vi "VI Properties Editor.vi"() -> ()   [LabVIEW 2023, in "VI Properties Editor.lvlib"]
doc: "Displays a window to add and edit properties of VIs in a streamlined way."
uses:
  VI Properties Editor.lvlib
  Tree Map/Tree Map/Tree Map.lvclass
  <vilib>/picture/picture.llb/imagedata.ctl
  CTLs/Main State Data.ctl
  CTLs/Control Properties.ctl
  CTLs/VI Properties.ctl
  CTLs/Main Front Panel Controls.ctl
  CTLs/Config.ctl
  <vilib>/Utility/miscctls.llb/LVSelectionTypeDef.ctl
  CTLs/Filter Type.ctl
  CTLs/Column Name.ctl
  CTLs/Filter Info.ctl
  CTLs/Confirmation Type.ctl
  CTLs/Main References.ctl
  CTLs/Sort Info.ctl
  CTLs/VI Data Map.ctl
  <vilib>/Utility/miscctls.llb/LVRowAndColumnTypeDef.ctl
  <vilib>/Utility/miscctls.llb/LVNodeAndColumnTypeDef.ctl
panel:
  in  "VI Tree":string(tree) caption="Select a VI to View/Edit Properties:"
  in  "Same Title as VI?":bool caption="Same as VI name"
  in  "Window Title":string
  in  "Add Copyright":bool
  out "Inline?":bool
  out "Reentrant?":bool
  in  "Set all VIs":bool
  in  "Help Tag":string
  in  "Help Path":string
  out "Path to VI":string
  in  "VI Description":string
  out "VI Connector Pane":picture
  in  "Controls":string[][](table)
  out "Current Filter":string
  out "Current Counts":string
  out "Current Source":string
  # "Controls"
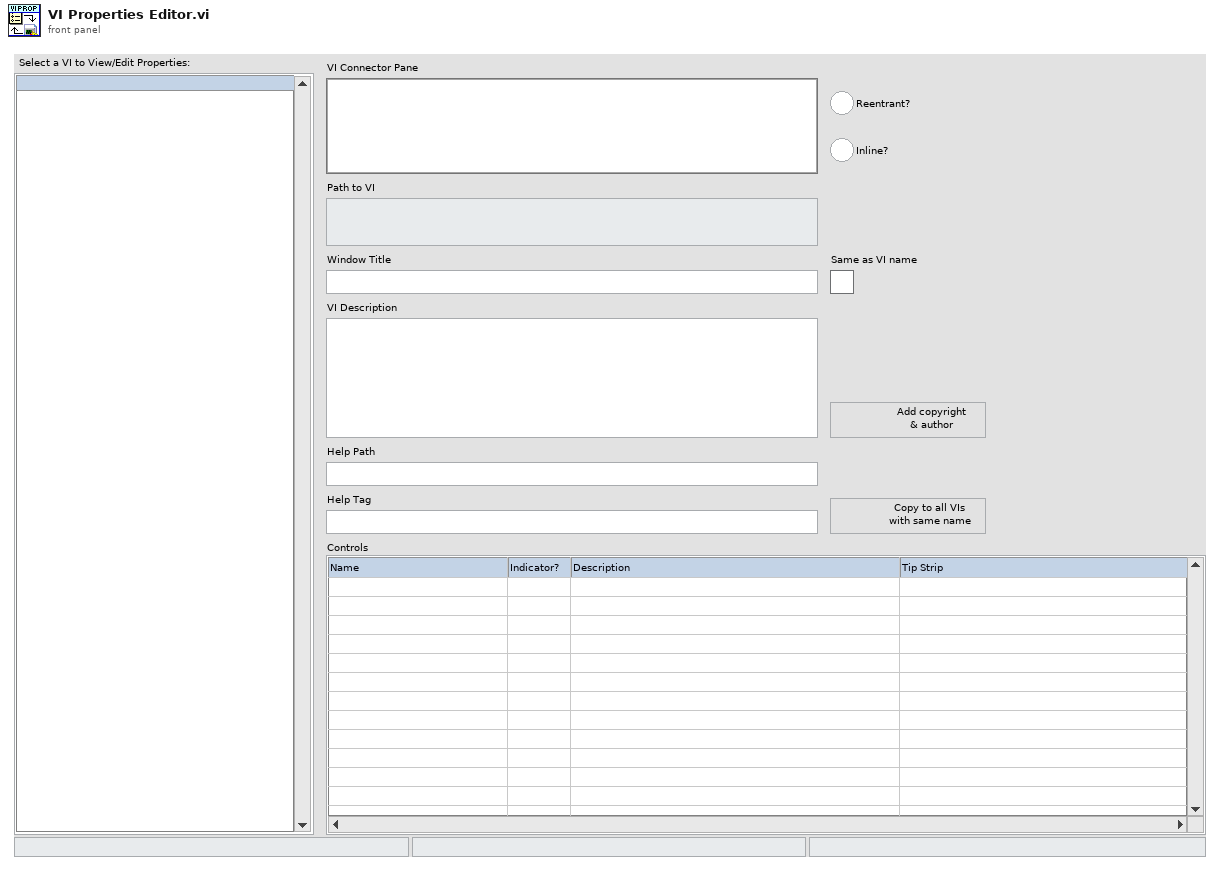
[diagram p1: front panel]
types:
  T1 = typedef "VI Properties Editor.lvlib/Main State Data.ctl" = cluster{"Core":cluster{"Current VI Reference":refnum<vi>, "Close Panel on Exit?":bool}, "FP Refs":T2, "New VI Data":T3, "Saved VI Data":T3, "Current Path":path, "FP":T7, "Config Path":path, "Config":T8, "Desc Selection":T12, "Displayed Hierarchies":string[], "Filter":T9, "Sort":T13, "Tree Map":refnum<class "Tree Map.lvclass">}
  T2 = typedef "VI Properties Editor.lvlib/Main References.ctl" = cluster{"VI Tree":refnum<vi>, "Window Title":refnum<vi>, "Same as VI?":refnum<vi>, "VI Desc":refnum<vi>, "Help Path":refnum<vi>, "Help Tag":refnum<vi>, "Controls":refnum<vi>}
  T3 = typedef "VI Properties Editor.lvlib/VI Data Map.ctl" = map{string, cluster{"VI":T4, "Ctl Properties":T6[]}}
  T4 = typedef "VI Properties Editor.lvlib/VI Properties.ctl" = cluster{"Name":string, "Path":path, "Type":enum32{"invalid VI type", "Standard VI", "Control VI", "Global VI", "Polymorphic VI", "Configuration VI", "SubSystem", "Facade VI", "Method VI", "Statechart Diagram VI"}, "Window Title":string, "Description":string, "Help Path":path, "Help Tag":string, "Custom Title?":bool, "Reentrant?":bool, "Inlined?":bool, "Conpane Img":T5}
  T5 = typedef "imagedata.ctl" = cluster{"image type":i32, "image depth":i32, "image":u8[], "mask":u8[], "colors":u32[], "Rectangle":cluster{"left":i16, "top":i16, "right":i16, "bottom":i16}}
  T6 = typedef "VI Properties Editor.lvlib/Control Properties.ctl" = cluster{"UID":i32, "Name":string, "Description":string, "Tip Strip":string, "Is Indicator?":bool, "Is on ConPane?":bool}
  T7 = typedef "VI Properties Editor.lvlib/Main Front Panel Controls.ctl" = cluster{"VI Selected":string, "Help Path":string, "Help Tag":string, "VI Desc":string, "Controls":string[][], "Window Title":string, "Same Title?":bool}
  T8 = typedef "VI Properties Editor.lvlib/Config.ctl" = cluster{"Copyright Path":path, "Recent Folders":path[], "Recent Files":path[], "Recent Filters":T9[], "Abbreviate Names?":bool, "Format Bold Tags?":bool, "Show ConPane Only?":bool, "Confirm Save?":bool, "Confirm Revert?":bool, "Confirm Save All?":bool, "Confirm Revert All?":bool, "Confirm Exit?":bool}
  T9 = typedef "VI Properties Editor.lvlib/Filter Info.ctl" = cluster{"Filter Column":T10, "Filter Type":T11, "Filter Value":string, "New Data?":bool, "Enabled?":bool}
  T10 = typedef "VI Properties Editor.lvlib/Column Name.ctl" = enum16{"Name", "Path", "Type", "Window Title", "Description", "Help Path", "Help Tag", "Custom Title?", "Reentrant?", "Inlined?"}
  T11 = typedef "VI Properties Editor.lvlib/Filter Type.ctl" = enum16{"Contains", "Equals", "Starts with", "Ends with", "Does not contain", "Does not equal", "Is empty", "Is not empty"}
  T12 = typedef "LVSelectionTypeDef.ctl" = cluster{"Selection Start":u32, "Selection End":u32}
  T13 = typedef "VI Properties Editor.lvlib/Sort Info.ctl" = cluster{"Sort Column":T10, "Ascending?":bool, "Enabled?":bool}
  T14 = enum32{"Invalid", "Standard", "Closed", "Hidden", "Minimized", "Maximized"}
  T15 = enum32{"invalid app kind", "Development System", "Run Time System", "Student Edition", "Embedded LabVIEW", "Evaluation", "Custom"}
  T16 = typedef "LVRowAndColumnTypeDef.ctl" = cluster{"Row":i32, "Column":i32}
  T17 = enum32{"invalid VI type", "Standard VI", "Control VI", "Global VI", "Polymorphic VI", "Configuration VI", "SubSystem", "Facade VI", "Method VI", "Statechart Diagram VI"}
  T18 = typedef "VI Properties Editor.lvlib/Confirmation Type.ctl" = enum16{"Save", "Revert", "Save All", "Revert All"}
  T19 = typedef "LVNodeAndColumnTypeDef.ctl" = cluster{"Node":string, "Column":i32}
  T20 = map{string, cluster{"VI":T4, "Ctl Properties":T6[]}}
  T21 = enum8{"Enabled", "Disabled", "Disabled and Grayed Out"}
  T22 = enum16{"Left Button", "Center Button", "Right Button", "Window Close"}
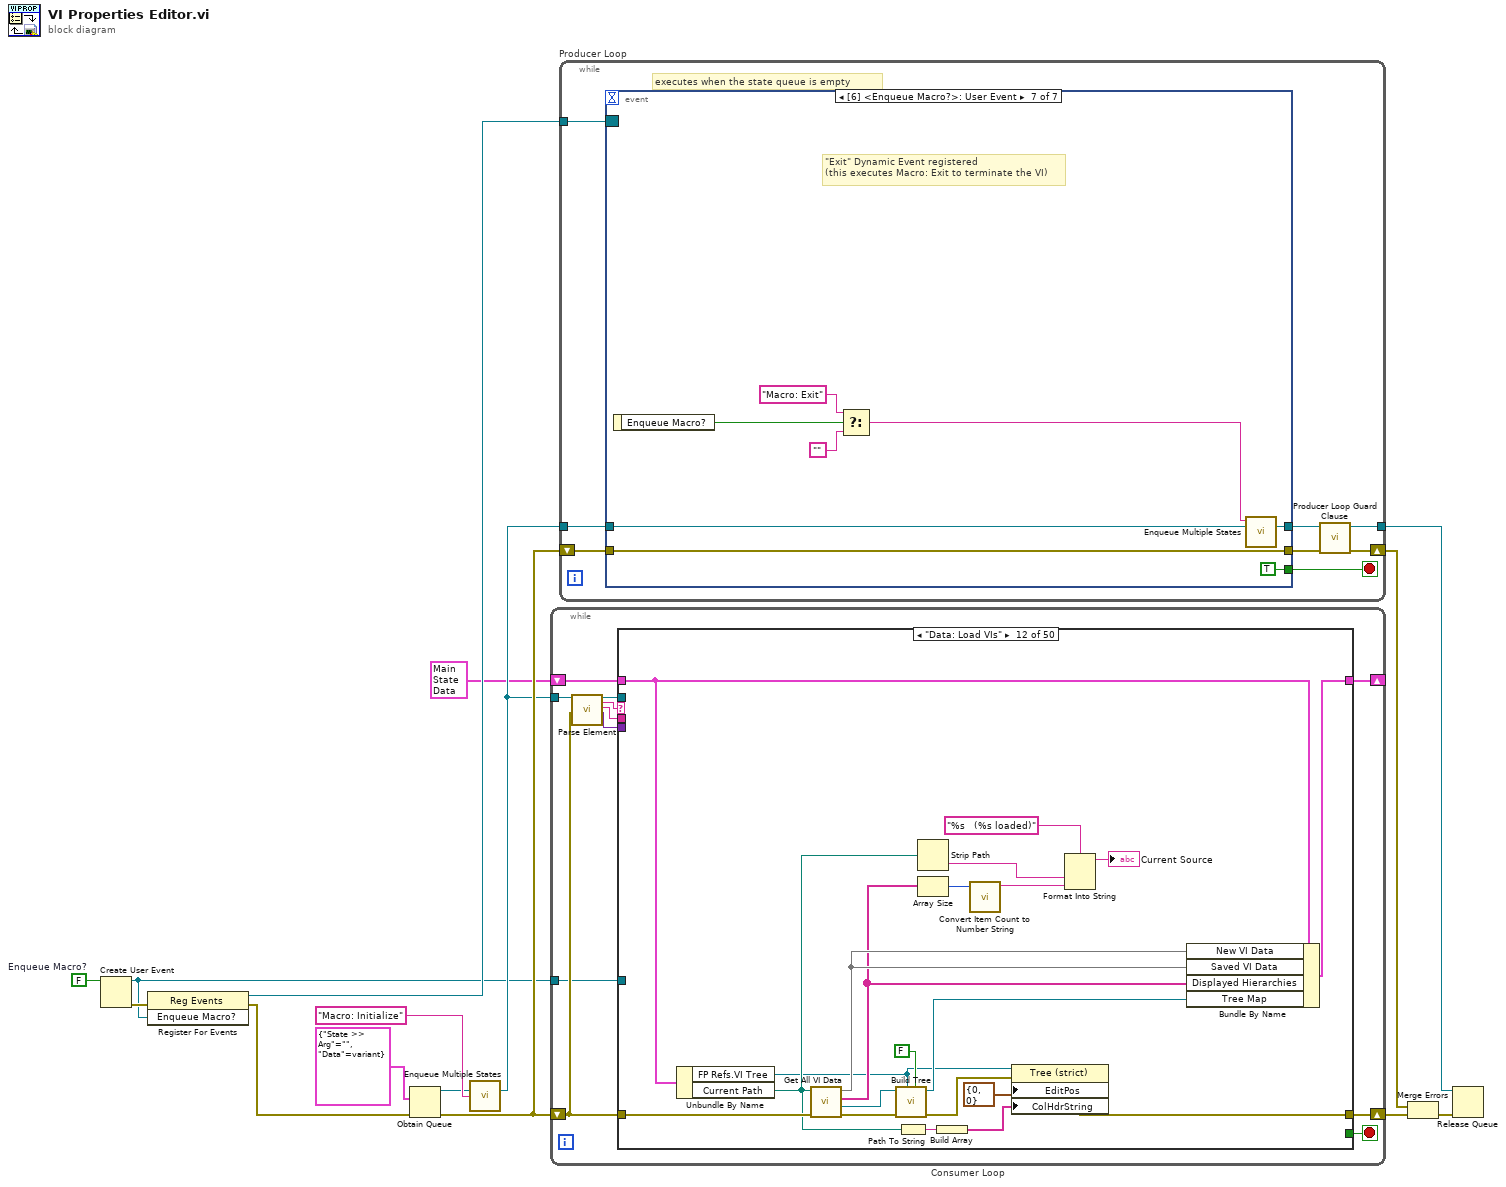
[diagram p0: block diagram]
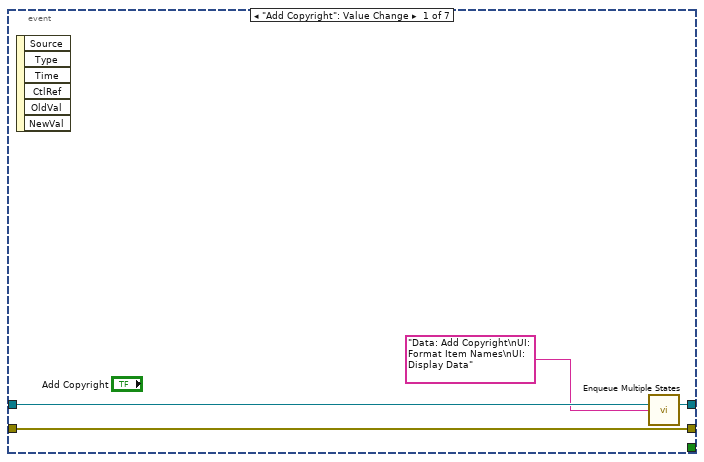
[diagram p2: hidden frame]
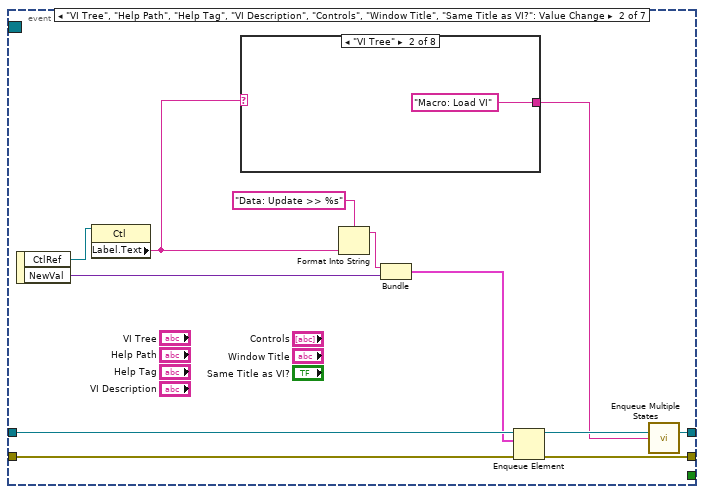
[diagram p3: hidden frame]
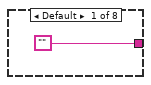
[diagram p4: hidden frame]
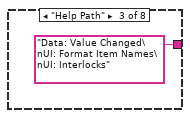
[diagram p5: hidden frame]
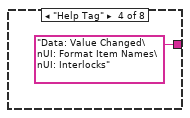
[diagram p6: hidden frame]
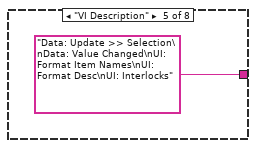
[diagram p7: hidden frame]
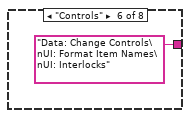
[diagram p8: hidden frame]
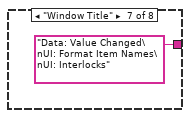
[diagram p9: hidden frame]
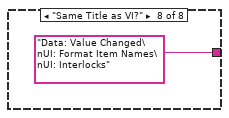
[diagram p10: hidden frame]
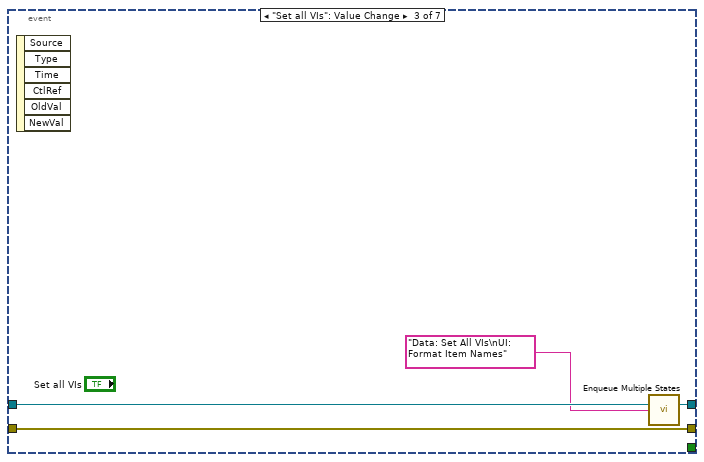
[diagram p11: hidden frame]
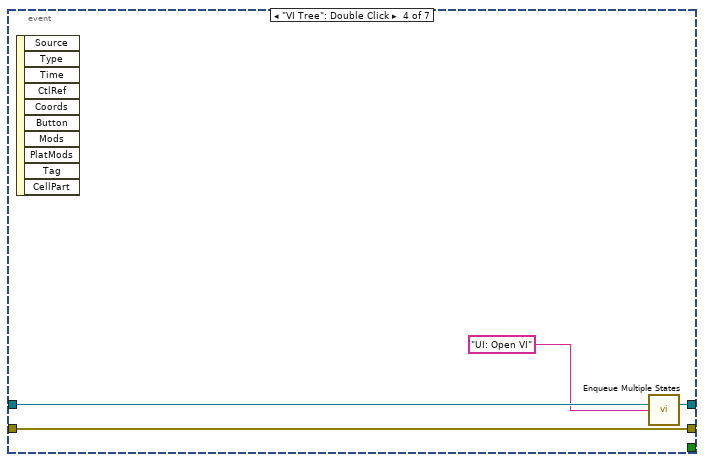
[diagram p12: hidden frame]
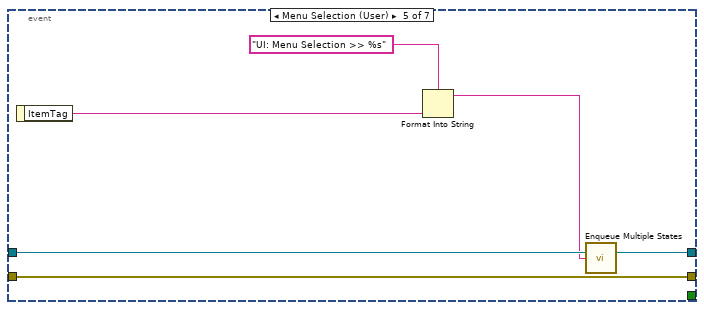
[diagram p13: hidden frame]
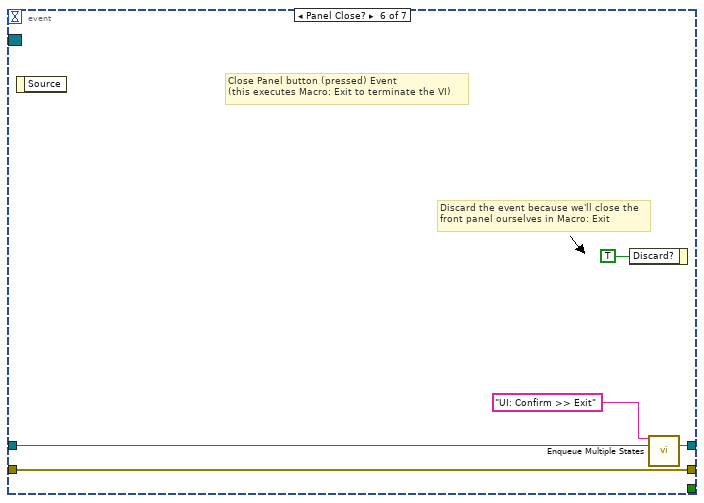
[diagram p14: hidden frame]
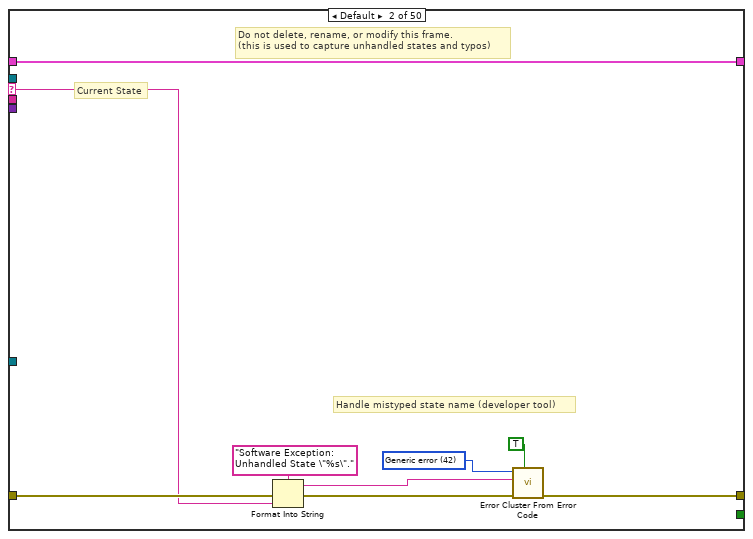
[diagram p16: hidden frame]
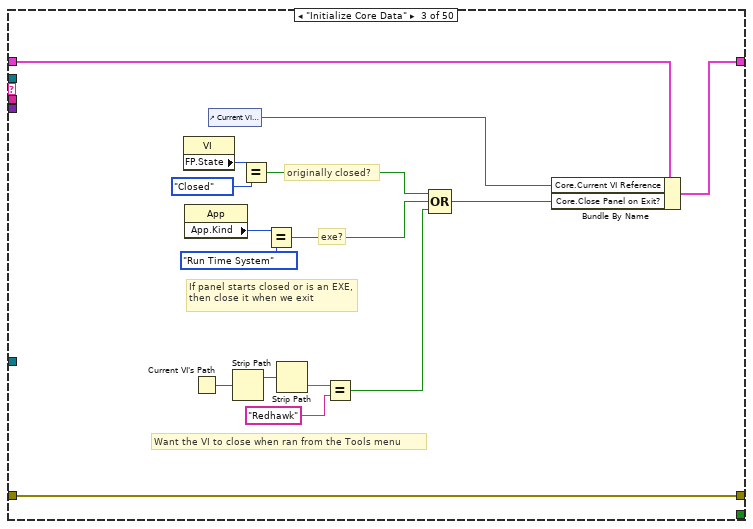
[diagram p17: hidden frame]
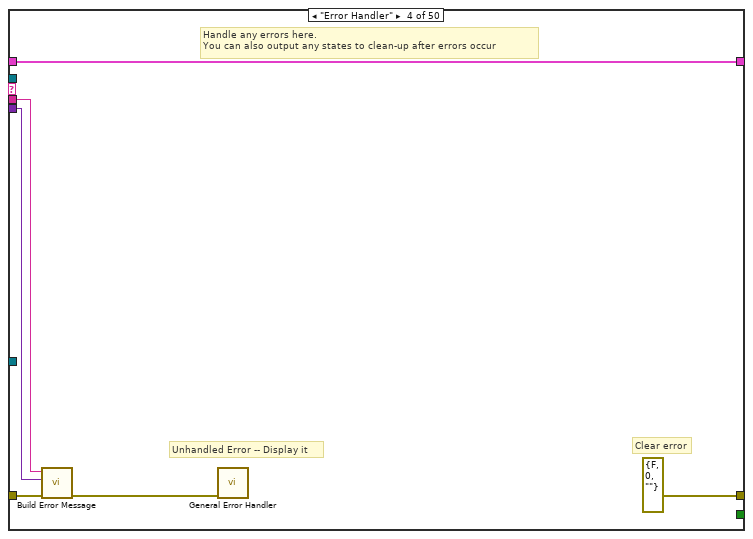
[diagram p18: hidden frame]
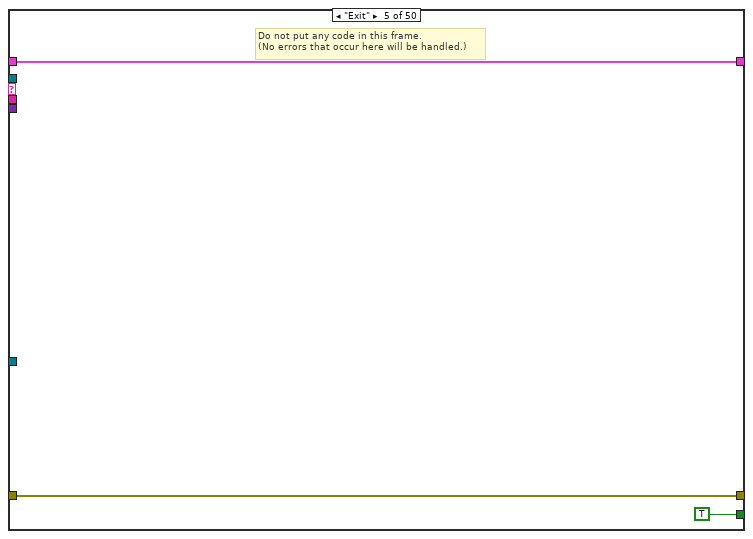
[diagram p19: hidden frame]
diagram:
  w5 = FALSE  # Enqueue Macro?
  n1 = Create User Event(user event datatype=w5) -> (user event=w2:refnum<user-event>, error out=w6:errorcluster)  [unwired: 1 in]
  n2 = register-events(error in=w6, w2) -> (reference out=w3:refnum<event-registration>, error out=w4:errorcluster)  [unwired: 1 in]
  n3 = Obtain Queue(element data type=cluster{"State >> Arg":string, "Data":variant} {"State >> Arg"="", "Data"=variant}, error in (no error)=w4) -> (queue out=w12:refnum<queue>, error out=w15:errorcluster)  [unwired: 3 in, 1 out]
  n4 = call "Enqueue Multiple States.vi"("queue in"=w12, "State(s) at Back"="Macro: Initialize") -> ("queue out"=w11:refnum<queue>)  [unwired: 13 in]
  n5 = while "Consumer Loop" {
    shift-right: [w23] -> _
    shift-left: T1 {"Core"={"Current VI Reference"=refnum, "Close Panel on Exit?"=FALSE}, "FP Refs"={"VI Tree"=refnum, "Window Title"=refnum, "Same as VI?"=refnum, "VI Desc"=refnum, "Help Path"=refnum, "Help Tag"=refnum, "Controls"=refnum}, "New VI Data"={}, "Saved VI Data"={}, "Current Path"=path "", "FP"={"VI Selected"="", "Help Path"="", "Help Tag"="", "VI Desc"="", "Controls"=[], "Window Title"="", "Same Title?"=FALSE}, "Config Path"=path "", "Config"={"Copyright Path"=path "", "Recent Folders"=[], "Recent Files"=[], "Recent Filters"=[], "Abbreviate Names?"=FALSE, "Format Bold Tags?"=FALSE, "Show ConPane Only?"=FALSE, "Confirm Save?"=FALSE, "Confirm Revert?"=FALSE, "Confirm Save All?"=FALSE, "Confirm Revert All?"=FALSE, "Confirm Exit?"=FALSE}, "Desc Selection"={"Selection Start"=0, "Selection End"=0}, "Displayed Hierarchies"=[], "Filter"={"Filter Column"=enum."Description", "Filter Type"=enum."Contains", "Filter Value"="", "New Data?"=FALSE, "Enabled?"=FALSE}, "Sort"={"Sort Column"=enum."Description", "Ascending?"=FALSE, "Enabled?"=FALSE}, "Tree Map"=refnum} ("VI Properties Editor State Data") -> [w22]
    shift-right: [w26] -> w10
    shift-left: w15 -> [w25]
    tunnel: w11 -> [w21]
    tunnel: w2 -> [w16]
    stop <- w24 stop-if-true
    n6 = call "Parse Element.vi"("queue in"=w21, "error in (no error)"=w25) -> ("queue out"=w20:refnum<queue>, "State"=w19:string, "Arg"=w18:string, "Data"=w17:variant)  [unwired: 14 in]
    n7 = case shown="\"Data: Load VIs\"" w19 {
      selector: w19 -> [_ w29 _ _ _ _ _ _ _ _ _ _ _ _ _ _ _ _ _ _ _ _ _ _ _ _ _ _ _ _ _ _ _ _ _ _ _ _ _ _ _ _ _ _ _ _ _ _ _ _]
      tunnel: w20 -> [_ _ _ _ _ _ _ _ _ w108 _ _ _ _ _ _ _ _ _ _ _ _ _ _ _ w250 _ _ _ _ _ _ w401 w433 _ _ _ _ _ _ w527 w648 w662 _ w671 w675 w683 w690 w697 w711]
      tunnel: w18 -> [_ _ _ w54 _ _ _ _ w93 _ _ _ _ _ _ _ _ _ _ _ w216 _ _ _ _ w245 w252 w260 w332 _ _ _ w388 w419 _ _ _ _ _ w485 w523 _ _ _ _ _ w679 w688 w695 _]
      tunnel: w22 -> [w27 w31 w48 w58 w61 w63 w77 w91 w95 w104 w111 w133 w138 w153 w162 w170 w176 w186 w196 w204 w219 w232 w236 w238 w241 w251 w253 w262 w337 w352 w365 w385 w399 w430 w437 w446 w457 w468 w476 w483 w524 w645 w659 w668 w672 w676 w684 w687 w694 w715]
      tunnel: [w28 w36 w53 errorcluster {"status"=FALSE, "code"=0, "source"=""} ("error out") w62 w64 w71 w89 w96 w106 w112 w114 w135 w154 w163 w171 w174 w183 w197 w205 w225 w234 w237 w239 w243 w248 w254 w263 w333 w343 w361 w383 w390 w431 w438 w447 w453 w464 w475 w488 w525 w646 w660 w669 w673 w677 w685 w686 w693 w707] -> w26
      tunnel: w25 -> [w28 w35 w53 w57 w62 w64 w70 w89 w97 w107 w113 w132 w136 w154 w163 w171 w175 w184 w197 w205 w221 w235 w237 w239 w244 w249 w255 w264 w334 w344 w361 w383 w392 w432 w439 w448 w454 w465 w480 w487 w526 w647 w661 w669 w673 w677 w685 w686 w693 w716]
      tunnel: [_ _ _ _ TRUE _ _ _ _ _ _ _ _ _ _ _ _ _ _ _ _ _ _ _ _ _ _ _ _ _ _ _ _ _ _ _ _ _ _ _ _ _ _ _ _ _ _ _ _ _] -> w24
      tunnel: [w27 w31 w52 w58 w61 w63 w76 w90 w94 w105 w111 w134 w137 w152 w161 w169 w173 w187 w198 w206 w224 w232 w236 w238 w241 w251 w253 w262 w337 w352 w365 w385 w398 w430 w437 w446 w456 w467 w476 w484 w522 w644 w658 w668 w672 w676 w684 w687 w694 w715] -> w23
      tunnel: w17 -> [_ _ _ w55 _ _ _ _ w92 _ _ _ _ _ _ _ _ _ _ _ _ _ _ _ _ _ _ _ _ _ _ _ _ _ _ _ _ _ _ _ _ _ _ _ _ _ _ _ _ _]
      tunnel: w16 -> [_ _ _ _ _ _ _ _ _ _ _ _ _ _ _ _ _ _ _ _ _ _ _ _ _ _ _ _ _ _ _ _ _ _ _ _ _ _ _ _ _ _ _ _ _ _ _ _ _ w706]
      frame "---------- Core ----------" {
        # "Do not put any code in this frame.\n(it is a separator no-op)"
      }
      frame Default {
        w33 = 42 items=["No error", "Argument error", "Memory is full", "Out of zone", "End of file", "File already open", "Generic file I/O error", "File not found", "File permission error", "Disk is full", "Duplicate path", "Too many files open", "System feature not enabled", "Resource file not found", "Cannot add resource", "Resource not found", "Image not found", "Image memory error", "Pen does not exist", "Config type invalid", "Config token not found", "Config parse error", "Config memory error", "Bad external code format", "Bad external code offset", "External code not present", "Null window", "Destroy window error", "Null menu", "Print aborted", "Bad print record", "Print driver error", "Windows error during printing", "Memory error during printing", "Print dialog error", "Generic print error", "Invalid device refnum", "Device not found", "Device parameter error", "Device unit error", "Cannot open device", "Device call aborted", "Generic error", "Cancelled by user", "Object ID too low", "Object ID too high", "Object not in heap", "Unknown heap", "Unknown object (invalid DefProc)", "Unknown object (DefProc not in table)", "Message out of range", "Invalid (null) method", "Unknown message", "Manager call not supported", "Bad address", "Network operation in progress", "Network operation timed out", "Connection is busy", "Network attribute not supported", "Network error", "Address in use", "System out of memory", "Connection aborted", "Connection refused", "Not connected", "Already connected", "Connection closed", "Initialization error (interapplication manager)", "Bad occurrence", "Wait on unbound occurrence handler", "Occurrence queue overflow", "Datalog type conflict", "Unused", "Unrecognized type (interapplication manager)", "Memory corrupt", "Failed to make temporary DLL", "Old CIN version", "Drag socket not found", "Failed to load drop-object", "Failed to register OLE object", "Failed to release OLE object", "Format specifier type mismatch", "Unknown format specifier", "Too few format specifiers", "Too many format specifiers", "Scan failed", "Newer CIN version", "Error converting to variant", "Runtime menu error", "Password tampered", "Variant attribute not found", "Incompatible variant data type", "Event data is not available", "Event Store is not present", "Occurrence is not found", "Event Queue is not created", "Event info is not available", "Refnum passed is NULL", "Error retrieving Class GUID", "Error retrieving CoClass GUID", "Error retrieving TypeLib GUID.", "Bad built application magic bytes.", "Specific driver is different from the specific driver associated with the Logical Name.", "There is no session opened to the class driver.", "Max Error", "MAX - Error with config objects", "MAX - Error loading configuration", "MAX - Group not supported"]
        # "Current State"
        # "Do not delete, rename, or modify this frame.\n(this is used to capture unhandled states and typos)"
        # "Handle mistyped state name (developer tool)"
        n8 = Format Into String(format string="Software Exception: Unhandled State \"%s\"." ("message"), error in=w35, w29) -> (resulting string=w32:string, error out=w37:errorcluster)  [unwired: 1 in]
        n9 = call <vilib>:"Error Cluster From Error Code.vi"("show call chain? (False)"=TRUE, "error in (no error)"=w37, "error message (\"\")"=w32, "error code (0)"=w33) -> ("error out"=w36:errorcluster)  [unwired: 5 in]
      }
      frame "Initialize Core Data" {
        # "Want the VI to close when ran from the Tools menu"
        # "originally closed?"
        # "exe?"
        # "If panel starts closed or is an EXE, then close it when we exit"
        n10 = property class="VI"() -> ("FP.State"=w45:T14)  [unwired: 2 in, 2 out]
        n11 = property class="App"() -> ("App.Kind"=w51:T15)  [unwired: 2 in, 2 out]
        n12 = Current VI's Path() -> (path=w42:path)
        n13 = control-ref of="Current VI Reference"() -> (w46:refnum<vi>)
        n14 = Strip Path(path=w42) -> (stripped path=w41:path)  [unwired: 1 out]
        n15 = Equal?(x=w45, y=T14."Closed" ("Front Panel Window:State")) -> (x = y?=w43:bool)
        n16 = Equal?(x=w51, y=T15."Run Time System" ("Application:Kind")) -> (x = y?=w49:bool)
        n17 = Strip Path(path=w41) -> (name=w40:string)  [unwired: 1 out]
        n18 = Equal?(x=w40, y="Redhawk" ("name")) -> (x = y?=w38:bool)
        n19 = Compound Arithmetic op=OR(w43, w49, w38) -> (w47:bool)
        n20 = Bundle By Name(cluster=w48, "Core.Current VI Reference"=w46, "Core.Close Panel on Exit?"=w47) -> (w52:T1)
      }
      frame "Error Handler" {
        # "Unhandled Error -- Display it"
        # "Handle any errors here.\nYou can also output any states to clean-up after errors occur"
        # "Clear error"
        n21 = call "Build Error Message.vi"("error in (no error)"=w57, "Data"=w55, "Arg"=w54) -> ("error out"=w56:errorcluster)  [unwired: 8 in]
        n22 = call <vilib>:"General Error Handler.vi"("error in (no error)"=w56) -> ()  [unwired: 10 in, 5 out]
      }
      frame "Exit" {
        # "Do not put any code in this frame.\n(No errors that occur here will be handled.)"
      }
      frame "---------- Data ----------" {
        # "Do not put any code in this frame.\n(It is a separator no-op. You can make a copy of this frame to create a new Data frame)"
      }
      frame "Data: Initialize" {
        # "Initialize the shift-register data, here."
        n23 = call "Config Path--constant.vi"() -> ("Config Path"=w66:path)  [unwired: 11 in]
        n24 = Strip Path(path=w66) -> (stripped path=w75:path)  [unwired: 1 out]
        n25 = call <vilib>:"Check if File or Folder Exists.vi"("error in (no error)"=w70, "path"=w75) -> ("error out"=w74:errorcluster, "file or folder exists?"=w72:bool, "dup path"=w73:path)  [unwired: 7 in]
        n26 = case shown="True" w72 {
          tunnel: [w80 w81] -> w71
          tunnel: w74 -> [w79 w81]
          tunnel: w73 -> [w78 _]
          frame False {
            n27 = Create Folder(path (use dialog)=w78, error in=w79) -> (error out=w80:errorcluster)  [unwired: 1 in, 2 out]
          }
          frame True {
          }
        }
        n28 = Bundle By Name(cluster=w77, "FP.VI Selected"="", "Sort.Sort Column"=Column_Name."Name" ("Sort Column"), "Sort.Ascending?"=TRUE ("Ascending?"), "Sort.Enabled?"=FALSE ("Ascending?"), "Config Path"=w66) -> (w76:T1)
      }
      frame "Data: Bundle Refs" {
        n29 = control-ref of="Window Title"() -> (w87:refnum<vi>)
        n30 = control-ref of="Same Title as VI?"() -> (w86:refnum<vi>)
        n31 = control-ref of="VI Description"() -> (w85:refnum<vi>)
        n32 = control-ref of="Help Path"() -> (w84:refnum<vi>)
        n33 = control-ref of="Help Tag"() -> (w83:refnum<vi>)
        n34 = control-ref of="Controls"() -> (w82:refnum<vi>)
        n35 = control-ref of="VI Tree"() -> (w88:refnum<vi>)
        n36 = Bundle By Name(cluster=w91, "FP Refs.VI Tree"=w88, "FP Refs.Window Title"=w87, "FP Refs.Same as VI?"=w86, "FP Refs.VI Desc"=w85, "FP Refs.Help Path"=w84, "FP Refs.Help Tag"=w83, "FP Refs.Controls"=w82) -> (w90:T1)
      }
      frame "Data: Update" {
        n37 = call "Update State Data.vi"("error in (no error)"=w97, "Data"=w92, "Argument"=w93, "State Data"=w95) -> ("error out"=w96:errorcluster, "State Data out"=w94:T1)  [unwired: 6 in]
      }
      frame "Data: Read Config" {
        n38 = Unbundle By Name(w104) -> ("Config Path"=w103:path)
        n39 = call "Read Config.vi"("error in (no error)"=w107, "Path"=w103) -> ("error out"=w106:errorcluster, "Config"=w102:T8, "File Created?"=w101:bool)  [unwired: 7 in]
        n40 = Bundle By Name(cluster=w104, "Config"=w102) -> (w105:T1)
        n41 = Select(t="Data: Write Config", s=w101, f="") -> (s? t:f=w98:string)
        n42 = call "Enqueue Multiple States.vi"("queue in"=w108, "State(s) at Back"=w98) -> ()  [unwired: 13 in, 1 out]
      }
      frame "Data: Write Config" {
        n43 = Unbundle By Name(w111) -> ("Config Path"=w109:path, "Config"=w110:T8)
        n44 = call "Write Config.vi"("error in (no error)"=w113, "Config"=w110, "Path"=w109) -> ("error out"=w112:errorcluster)  [unwired: 8 in]
      }
      frame "Data: Load VIs" {
        n45 = Unbundle By Name(w133) -> ("FP Refs.VI Tree"=w118:refnum<vi>, "Current Path"=w122:path)
        n46 = call "Get All VI Data.vi"("error in (no error)"=w132, "Path"=w122) -> ("error out"=w120:errorcluster, "Tree Map out"=w124:refnum<class "Tree Map.lvclass">, "Displayed Hierarchies"=w129:string[], "VI Data Map"=w131:T3)  [unwired: 6 in]
        n47 = call "Build Tree.vi"("Defer Updates (T)"=FALSE ("Defer Updates"), "Tree"=w118, "error in (no error)"=w120, "Tree Map in"=w124) -> ("error out"=w115:errorcluster, "Tree Map out"=w119:refnum<class "Tree Map.lvclass">)  [unwired: 6 in]
        n48 = Path To String(path=w122) -> (string=w121:string)
        n49 = Strip Path(path=w122) -> (name=w127:string)  [unwired: 1 out]
        n50 = Array Size(array=w129) -> (size(s)=w126:i32)
        n51 = Build Array(w121) -> (w117:string[])
        n52 = call "Convert Item Count to Number String.vi"("Item Count"=w126) -> ("Number of Items String"=w125:string)  [unwired: 10 in]
        n53 = property class="Tree (strict)"(reference=w118, error in=w115, "EditPos"=T16 {"Row"=0, "Column"=0} ("Edit Position"), "ColHdrString"=w117) -> (error out=w114:errorcluster)  [unwired: 1 out]
        n54 = Format Into String(format string="%s   (%s loaded)", w127, w125) -> (resulting string=→"Current Source":string)  [unwired: 2 in, 1 out]
        n55 = Bundle By Name(cluster=w133, "New VI Data"=w131, "Saved VI Data"=w131, "Displayed Hierarchies"=w129, "Tree Map"=w119) -> (w134:T1)
      }
      frame "Data: Filter/Sort VIs" {
        n56 = in-place {
          in-place-border: w136 -> [w145]
          in-place-border: [w144] -> w135
          n57 = in-place-cluster #1(w138) -> ("Sort"=w149:T13, "Filter"=w150:T9, "Saved VI Data"=w140:T3, "New VI Data"=w141:T3)  [unwired: 1 out]
          n58 = call "Filter and Sort Items.vi"("Sort Info"=w149, "Filter Info"=w150, "error in"=w145, "New VI Data"=w141, "Saved VI Data"=w140) -> ("error out"=w144:errorcluster, "Displayed Hierarchies"=w143:string[], "New VI Data out"=w142:T3, "Saved VI Data out"=w139:T3)  [unwired: 3 in]
          n59 = call "Convert Filter to Display String.vi"("Filter Info"=w150) -> ("String"=w146:string)  [unwired: 10 in]
          n60 = Concatenate Strings("Current filter:  " ("string"), w146) -> (→"Current Filter":string)
          n61 = in-place-cluster #1("Sort"=w149, "Filter"=w150, "Saved VI Data"=w139, "New VI Data"=w142, "Displayed Hierarchies"=w143) -> (w137:T1)
        }
      }
      frame "Data: Value Changed" {
        n62 = Unbundle By Name(w153) -> ("FP"=w151:T7)
        n63 = in-place {
          in-place-border: w151 -> [w156]
          n64 = in-place-cluster #2(w153) -> ("New VI Data"=w155:T3)
          n65 = call "Set VI Properties.vi"("Front Panel Controls"=w156, "VI Data Map"=w155) -> ("VI Data Map out"=w157:T3)  [unwired: 9 in]
          n66 = in-place-cluster #2("New VI Data"=w157) -> (w152:T1)
        }
      }
      frame "Data: Revert Current" {
        n67 = Unbundle By Name(w162) -> ("FP.VI Selected"=w159:string, "Saved VI Data"=w160:T3)
        n68 = Look In Map(map=w160, key=w159) -> (value=w158:cluster{"VI":T4, "Ctl Properties":T6[]})  [unwired: 1 in, 1 out]
        n69 = in-place {
          in-place-border: w159 -> [w165]
          in-place-border: w158 -> [w164]
          n70 = in-place-cluster #3(w162) -> ("New VI Data"=w167:T3)
          n71 = Insert Into Map(map in=w167, key=w165, value=w164) -> (map out=w166:T3)  [unwired: 2 out]
          n72 = in-place-cluster #3("New VI Data"=w166) -> (w161:T1)
        }
      }
      frame "Data: Revert All" {
        n73 = Unbundle By Name(w170) -> ("Saved VI Data"=w168:T3)
        n74 = in-place {
          in-place-border: w168 -> [w172]
          n75 = in-place-cluster #4(w170) -> ()  [unwired: 1 out]
          n76 = in-place-cluster #4("New VI Data"=w172) -> (w169:T1)
        }
      }
      frame "Data: Save All" {
        n77 = in-place {
          in-place-border: w175 -> [w182]
          in-place-border: [w181] -> w174
          n78 = in-place-cluster #5(w176) -> ("New VI Data"=w178:T3, "Saved VI Data"=w177:T3)
          n79 = call "Save All VI Data.vi"("error in"=w182, "Saved VI Data"=w177, "New VI Data"=w178) -> ("error out"=w181:errorcluster, "Saved VI Data out"=w179:T3, "New VI Data out"=w180:T3)  [unwired: 6 in]
          n80 = in-place-cluster #5("New VI Data"=w180, "Saved VI Data"=w179) -> (w173:T1)
        }
      }
      frame "Data: Save Current" {
        n81 = Unbundle By Name(w186) -> ("FP.VI Selected"=w185:string)
        n82 = in-place {
          in-place-border: w185 -> [w189]
          in-place-border: w184 -> [w195]
          in-place-border: [w194] -> w183
          n83 = in-place-cluster #6(w186) -> ("New VI Data"=w190:T3, "Saved VI Data"=w193:T3)
          n84 = Look In Map(map=w190, key=w189) -> (value=w188:cluster{"VI":T4, "Ctl Properties":T6[]})  [unwired: 1 in, 1 out]
          n85 = node(w189, w188) -> (w191:T20)
          n86 = call "Save All VI Data.vi"("error in"=w195, "Saved VI Data"=w193, "New VI Data"=w191) -> ("error out"=w194:errorcluster, "Saved VI Data out"=w192:T3)  [unwired: 6 in, 1 out]
          n87 = in-place-cluster #6("New VI Data"=w190, "Saved VI Data"=w192) -> (w187:T1)
        }
      }
      frame "Data: Set All VIs" {
        n88 = in-place {
          n89 = in-place-cluster #7(w196) -> ("FP"=w199:T7, "New VI Data"=w201:T3)
          n90 = call "Copy to Matching Items.vi"("Front Panel Controls"=w199, "VI Data"=w201) -> ("VI Data out"=w200:T3)  [unwired: 9 in]
          n91 = in-place-cluster #7("FP"=w199, "New VI Data"=w200) -> (w198:T1)
        }
      }
      frame "Data: Change Controls" {
        n92 = Unbundle By Name(w204) -> ("FP.Controls"=w203:string[][], "FP.VI Selected"=w202:string)
        n93 = in-place {
          in-place-border: w203 -> [w209]
          in-place-border: w202 -> [w207]
          n94 = in-place-cluster #8(w204) -> ("New VI Data"=w210:T3)
          n95 = call "Set Control Properties.vi"("Selected VI"=w207, "Controls"=w209, "VI Data"=w210) -> ("VI Data out"=w208:T3)  [unwired: 8 in]
          n96 = in-place-cluster #8("New VI Data"=w208) -> (w206:T1)
        }
      }
      frame "Data: Add Copyright" {
        n97 = Unbundle By Name(w219) -> ("FP.VI Selected"=w213:string, "Config.Copyright Path"=w218:path)
        n98 = Read from Text File(file (use dialog)=w218, error in=w221) -> (refnum out=w222:refnum<file>, text=w217:string, error out=w223:errorcluster)  [unwired: 2 in, 1 out]
        n99 = Equal?(x=w216, y="All") -> (x = y?=w214:bool)
        n100 = Close File(refnum=w222, error in=w223) -> (error out=w220:errorcluster)  [unwired: 1 out]
        n101 = Select(t="", s=w214, f=w213) -> (s? t:f=w211:string)
        n102 = in-place {
          in-place-border: w220 -> [w230]
          in-place-border: [w229] -> w225
          in-place-border: w211 -> [w227]
          in-place-border: w217 -> [w226]
          n103 = in-place-cluster #9(w219) -> ("New VI Data"=w231:T3)
          n104 = call "Add Copyright.vi"("error in (no error)"=w230, "Copyright Text"=w226, "VI Selected"=w227, "VI Data Map"=w231) -> ("error out"=w229:errorcluster, "VI Data Map out"=w228:T3)  [unwired: 6 in]
          n105 = in-place-cluster #9("New VI Data"=w228) -> (w224:T1)
        }
      }
      frame "Data: Cleanup" {
        # "Cleanup any data and references, here.\n(this is called automatically, by the Macro: Exit)"
        n106 = Unbundle By Name(w232) -> ("Core.Current VI Reference"=w233:refnum<vi>)
        n107 = Close Reference(reference=w233, error in (no error)=w235) -> (error out=w234:errorcluster)
      }
      frame "---------- UI ----------" {
        # "Do not put any code in this frame.\n(It is a separator no-op. You can make a copy of this frame to create a new UI frame)"
      }
      frame "UI: Initialize" {
        # "Initialize the User Interface, here.\n(this is called automatically, by the Macro: Init)"
      }
      frame "UI: Initialize Menu" {
        n108 = Unbundle By Name(w241) -> ("Config"=w240:T8)
        n109 = Current VI's Menubar() -> (w242:refnum<k9>)
        n110 = call "Initialize Menu Items.vi"("error in (no error)"=w244, "Config"=w240, "Menu Ref"=w242) -> ("error out"=w243:errorcluster)  [unwired: 8 in]
      }
      frame "UI: Menu Selection" {
        n111 = Current VI's Menubar() -> (w246:refnum<k9>)
        n112 = call "Process Menu Selection.vi"("error in (no error)"=w249, "Argument"=w245, "Menu Ref"=w246) -> ("error out"=w248:errorcluster, "State(s) to Enqueue"=w247:string)  [unwired: 7 in]
        n113 = call "Enqueue Multiple States.vi"("queue in"=w250, "State(s) at Back"=w247) -> ()  [unwired: 13 in, 1 out]
      }
      frame "UI: Cursor Set" {
        # "Argument"
        # "Set and Unset Cursor Busy.\n(Usage: \"UI: Cursor Set >> Busy|Idle\")"
        n114 = case shown="\"Idle\", Default" w252 {
          tunnel: w255 -> [w257 w259]
          tunnel: [w256 w258] -> w254
          frame "Idle", Default {
            n115 = call <vilib>:"Unset Busy.vi"("error in (no error)"=w257) -> ("error out"=w256:errorcluster)  [unwired: 10 in]
          }
          frame "Busy" {
            n116 = call <vilib>:"Set Busy.vi"("error in (no error)"=w259) -> ("error out"=w258:errorcluster)  [unwired: 9 in, 1 out]
          }
        }
      }
      frame "UI: Front Panel State" {
        # "Argument"
        # "Set Front Panel Open or Closed\n(Usage: \"UI: Front Panel State >> Open|Close\")"
        n117 = Unbundle By Name(w262) -> ("Core.Current VI Reference"=w261:refnum<vi>)
        n118 = case shown="\"Open\", \"Standard\", Default" w260 {
          tunnel: w264 -> [w271 w285 w297 w310 w323]
          tunnel: [w272 w286 w298 w311 w324] -> w263
          tunnel: w261 -> [w269 w283 w295 w308 w321]
          frame "Open", "Standard", Default {
            w265 = T14."Standard" ("State")
            n119 = property class="VI"(reference=w269, error in=w271) -> (reference out=w268:refnum<vi>, error out=w270:errorcluster, "FP.State"=w267:T14)
            n120 = Not Equal?(x=w267, y=w265) -> (x != y?=w266:bool)
            n121 = case shown="False" w266 {
              tunnel: [w277 w278] -> w272
              tunnel: w270 -> [w276 w278]
              tunnel: w268 -> [w274 _]
              tunnel: w265 -> [w273 _]
              frame True {
                n122 = invoke class="VI" method="FP.Open"(reference=w274, error in=w276, "Activate"=TRUE, "State"=w273) -> (error out=w277:errorcluster)  [unwired: 1 in, 4 out]
              }
              frame False {
              }
            }
          }
          frame "Close", "Closed" {
            n123 = property class="VI"(reference=w283, error in=w285) -> (reference out=w282:refnum<vi>, error out=w284:errorcluster, "FP.State"=w280:T14)
            n124 = Not Equal?(x=w280, y=T14."Closed" ("Front Panel Window:State")) -> (x != y?=w279:bool)
            n125 = case shown="True" w279 {
              tunnel: [w287 w290] -> w286
              tunnel: w284 -> [w287 w289]
              tunnel: w282 -> [_ w288]
              frame False {
              }
              frame True {
                n126 = invoke class="VI" method="FP.Close"(reference=w288, error in=w289) -> (error out=w290:errorcluster)  [unwired: 1 in, 2 out]
              }
            }
          }
          frame "Hidden", "Hide" {
            w291 = T14."Hidden" ("State")
            n127 = property class="VI"(reference=w295, error in=w297) -> (reference out=w294:refnum<vi>, error out=w296:errorcluster, "FP.State"=w293:T14)
            n128 = Not Equal?(x=w293, y=w291) -> (x != y?=w292:bool)
            n129 = case shown="True" w292 {
              tunnel: [w302 w303] -> w298
              tunnel: w296 -> [w301 w303]
              tunnel: w294 -> [w300 _]
              tunnel: w291 -> [w299 _]
              frame True {
                n130 = invoke class="VI" method="FP.Open"(reference=w300, error in=w301, "State"=w299) -> (error out=w302:errorcluster)  [unwired: 2 in, 4 out]
              }
              frame False {
              }
            }
          }
          frame "Minimize", "Minimized" {
            w304 = T14."Minimized" ("State")
            n131 = property class="VI"(reference=w308, error in=w310) -> (reference out=w307:refnum<vi>, error out=w309:errorcluster, "FP.State"=w306:T14)
            n132 = Not Equal?(x=w306, y=w304) -> (x != y?=w305:bool)
            n133 = case shown="True" w305 {
              tunnel: [w315 w316] -> w311
              tunnel: w309 -> [w314 w316]
              tunnel: w307 -> [w313 _]
              tunnel: w304 -> [w312 _]
              frame True {
                n134 = invoke class="VI" method="FP.Open"(reference=w313, error in=w314, "State"=w312) -> (error out=w315:errorcluster)  [unwired: 2 in, 4 out]
              }
              frame False {
              }
            }
          }
          frame "Maximize", "Maximized" {
            w317 = T14."Maximized" ("State")
            n135 = property class="VI"(reference=w321, error in=w323) -> (reference out=w320:refnum<vi>, error out=w322:errorcluster, "FP.State"=w319:T14)
            n136 = Not Equal?(x=w319, y=w317) -> (x != y?=w318:bool)
            n137 = case shown="True" w318 {
              tunnel: [w328 w329] -> w324
              tunnel: w322 -> [w327 w329]
              tunnel: w320 -> [w326 _]
              tunnel: w317 -> [w325 _]
              frame True {
                n138 = invoke class="VI" method="FP.Open"(reference=w326, error in=w327, "State"=w325) -> (error out=w328:errorcluster)  [unwired: 2 in, 4 out]
              }
              frame False {
              }
            }
          }
        }
      }
      frame "UI: Panel Updates" {
        n139 = Unbundle By Name(w337) -> ("Core.Current VI Reference"=w336:refnum<vi>)
        n140 = Equal?(x=w332, y="Defer") -> (x = y?=w330:bool)
        n141 = property class="VI"(reference=w336, error in=w334) -> (error out=w338:errorcluster, "Panel"=w335:refnum<vi>)  [unwired: 1 out]
        n142 = property class="Pnl"(reference=w335, error in=w338, "Defer Panel Updates"=w330) -> (error out=w333:errorcluster)  [unwired: 1 out]
      }
      frame "UI: Interlocks" {
        n143 = Unbundle By Name(w352) -> ("New VI Data"=w342:T3, "FP.VI Selected"=w341:string)
        n144 = Look In Map(map=w342, key=w341) -> (value=w351:cluster{"VI":T4, "Ctl Properties":T6[]})  [unwired: 1 in, 1 out]
        n145 = Not Equal?(x="", y=w341) -> (x != y?=w340:bool)
        n146 = Unbundle By Name(w351) -> ("VI.Type"=w350:T17)
        n147 = Current VI's Menubar() -> (w345:refnum<k9>)
        n148 = call "UI Interlocks.vi"("Menu Ref"=w345, "error in (no error)"=w344, "VI Selected"=w341, "New VI Data"=w342) -> ("error out"=w343:errorcluster)  [unwired: 7 in]
        n149 = Not Equal?(x=w350, y=T17."Polymorphic VI" ("x")) -> (x != y?=w348:bool)
        n150 = call "Gray if False.vi"("Grayed Out?"=w340) -> ("Enabled State"=w346:T21)  [unwired: 10 in]
        n151 = call "Gray if False.vi"("Grayed Out?"=w348) -> ("Enabled State"=w347:T21)  [unwired: 10 in]
        n152 = property on="Set all VIs" class="Bool"("DisabledEnum"=w346) -> ()  [unwired: 2 in, 2 out]
        n153 = property on="Add Copyright" class="Bool"("DisabledEnum"=w346) -> ()  [unwired: 2 in, 2 out]
        n154 = property on="Controls" class="Tbl (strict)"("DisabledEnum"=w347) -> ()  [unwired: 2 in, 2 out]
      }
      frame "UI: Format Item Names" {
        # "#Todo"
        n155 = Unbundle By Name(w365) -> ("Displayed Hierarchies"=w359:string[], "Config.Abbreviate Names?"=w362:bool, "New VI Data"=w364:T3, "Saved VI Data"=w363:T3)
        n156 = call "Format Item Names.vi"("Displayed Hierarchies"=w359, "Abbreviate Names?"=w362, "Saved VI Data"=w363, "New VI Data"=w364) -> ("Number of Modified Items"=w355:i32)  [unwired: 6 in, 1 out]
        n157 = Array Size(array=w359) -> (size(s)=w357:i32)
        n158 = call "Convert Item Count to Number String.vi"("Item Count"=w357) -> ("Number of Items String"=w356:string)  [unwired: 10 in]
        n159 = call "Convert Item Count to Number String.vi"("Item Count"=w355) -> ("Number of Items String"=w354:string)  [unwired: 10 in]
        n160 = property on="VI Tree" class="Tree (strict)"("Value"="") -> ()  [unwired: 2 in, 2 out]
        n161 = Format Into String(format string="%s shown  -  %s modified", w356, w354) -> (resulting string=→"Current Counts":string)  [unwired: 2 in, 1 out]
      }
      frame "UI: Display Data" {
        n162 = Unbundle By Name(w385) -> ("Config.Show ConPane Only?"=w368:bool, "New VI Data"=w367:T3, "FP.VI Selected"=w366:string)
        n163 = Look In Map(map=w367, key=w366) -> (value=w384:cluster{"VI":T4, "Ctl Properties":T6[]})  [unwired: 1 in, 1 out]
        n164 = Unbundle By Name(w384) -> ("Ctl Properties"=w369:T6[], "VI.Window Title"=w375:string, "VI.Description"=w380:string, "VI.Help Path"=w379:path, "VI.Help Tag"=w377:string, "VI.Custom Title?"=w374:bool, "VI.Path"=w372:path, "VI.Reentrant?"=→"Reentrant?":bool, "VI.Inlined?"=→"Inline?":bool, "VI.Conpane Img"=w376:T5)
        n165 = Path To String(path=w379) -> (string=w378:string)
        n166 = Not(x=w374) -> (.not. x?=w373:bool)
        n167 = call "Convert Controls to Arrays.vi"("ConPane Only?"=w368, "Ctl Properties"=w369) -> ("Control Array"=w382:string[][])  [unwired: 9 in]
        n168 = Path To String(path=w372) -> (string=→"Path to VI":string)
        n169 = call <vilib>:"Draw Flattened Pixmap.vi"("image data"=w376) -> ("new picture"=→"VI Connector Pane":picture)  [unwired: 8 in]
        n170 = local write "Controls"(w382) -> ()
        n171 = local write "Window Title"(w375) -> ()
        n172 = local write "VI Description"(w380) -> ()
        n173 = local write "Help Path"(w378) -> ()
        n174 = local write "Help Tag"(w377) -> ()
        n175 = local write "Same Title as VI?"(w373) -> ()
      }
      frame "UI: Select Source" {
        # "catch cancel error"
        n176 = case shown="\"File\"" w388 {
          tunnel: [_ w405 w411] -> w400
          tunnel: [_ w404 w410] -> w397
          tunnel: [TRUE ("cancelled") w403 w409] -> w396
          frame Default {
          }
          frame "Folder" {
            n177 = call "File Dialog"("prompt"="Select the directory of VIs to update") -> ("selected path"=w404:path, "cancelled"=w403:bool, "error out"=w405:errorcluster)  [unwired: 11 in, 1 out]
          }
          frame "File" {
            n178 = call "File Dialog2"("prompt"="Select the project, library, or class VIs to update", "pattern (all files)"="*.lvproj;*.lvlib;*.lvclass", "pattern label"="Project, Library, or Class") -> ("selected path"=w410:path, "cancelled"=w409:bool, "error out"=w411:errorcluster)  [unwired: 9 in, 1 out]
          }
        }
        n179 = Format Into String(format string="UI: Cursor Set >> Busy\nData: Load VIs\nData: Update >> Reset Listbox\nData: Update >> %s Config\nData: Write Config\nUI: Initialize Menu\nData: Filter/Sort VIs\nMacro: Load VI\nUI: Format Item Names\nUI: Cursor Set >> Idle", w388) -> (resulting string=w387:string)  [unwired: 2 in, 1 out]
        n180 = Select(t="", s=w396, f=w387) -> (s? t:f=w394:string)
        n181 = call <vilib>:"Clear Errors.vi"("error in (no error)"=w400, "specific error code to clear (0: all)"=43) -> ("error out"=w391:errorcluster)  [unwired: 4 in, 1 out]
        n182 = call "Enqueue Multiple States.vi"("queue in"=w401, "State(s) at Back"=w394) -> ()  [unwired: 13 in, 1 out]
        n183 = Merge Errors(w392, w391) -> (w390:errorcluster)
        n184 = Bundle By Name(cluster=w399, "Current Path"=w397) -> (w398:T1)
      }
      frame "UI: Check Source" {
        n185 = Unbundle By Name(w430) -> ("Config.Recent Folders"=w424:path[], "Config.Recent Files"=w423:path[])
        n186 = Match Pattern(string=w419, regular expression="_") -> (before substring=w427:string, after substring=w428:string)  [unwired: 1 in, 2 out]
        n187 = Decimal String To Number(string=w428) -> (number=w421:i32)  [unwired: 2 in, 1 out]
        n188 = Equal?(x="FOLDER", y=w427) -> (x = y?=w425:bool)
        n189 = Select(t=w424, s=w425, f=w423) -> (s? t:f=w422:path[])
        n190 = Index Array(array=w422, index=w421) -> (element=w420:path)
        n191 = call <vilib>:"Check if File or Folder Exists.vi"("error in (no error)"=w432, "path"=w420) -> ("error out"=w431:errorcluster, "file or folder exists?"=w418:bool)  [unwired: 7 in, 1 out]
        n192 = Append True/False String(1:w418, 2:"Data: Update >> REM-%s\nData: Write Config\nUI: Initialize Menu", 3:"Macro: Load Recent Source >> %s") -> (0:w414:string)  [unwired: 1 in]
        n193 = Not(x=w418) -> (.not. x?=w417:bool)
        n194 = Format Into String(format string=w414, w419) -> (resulting string=w413:string)  [unwired: 2 in, 1 out]
        n195 = call "Source not Found"("Enable"=w417) -> ()  [unwired: 9 in, 2 out]
        n196 = call "Enqueue Multiple States.vi"("queue in"=w433, "State(s) at Back"=w413) -> ()  [unwired: 13 in, 1 out]
      }
      frame "UI: Open VI" {
        # "Open VI on DoubleClick"
        n197 = Unbundle By Name(w437) -> ("New VI Data"=w435:T3, "FP.VI Selected"=w434:string)
        n198 = Look In Map(map=w435, key=w434) -> (value=w444:cluster{"VI":T4, "Ctl Properties":T6[]})  [unwired: 1 in, 1 out]
        n199 = Unbundle By Name(w444) -> ("VI.Path"=w436:path)
        n200 = Open VI Reference(vi path=w436, error in (no error)=w439) -> (vi reference=w441:refnum<vi>, error out=w440:errorcluster)  [unwired: 4 in]
        n201 = invoke class="VI" method="FP.Open"(reference=w441, error in=w440) -> (reference out=w443:refnum<vi>, error out=w442:errorcluster)  [unwired: 3 in, 3 out]
        n202 = Close Reference(reference=w443, error in (no error)=w442) -> (error out=w438:errorcluster)
      }
      frame "UI: Edit Copyright" {
        n203 = Unbundle By Name(w446) -> ("Config.Copyright Path"=w445:path)
        n204 = Format Into String(format string="Notepad.exe %s", error in=w448, w445) -> (resulting string=w451:string, error out=w452:errorcluster)  [unwired: 1 in]
        n205 = call <vilib>:"System Exec.vi"("wait until completion? (T)"=FALSE, "error in (no error)"=w452, "command line"=w451) -> ("error out"=w447:errorcluster)  [unwired: 5 in, 3 out]
      }
      frame "UI: Add Bold Tags" {
        n206 = control-ref of="VI Description"() -> (w462:refnum<vi>)
        n207 = property class="Str"(reference=w462, error in=w454) -> (reference out=w459:refnum<vi>, error out=w463:errorcluster, "Value"=w461:string, "Text.Selection"=w460:T12)
        n208 = call "Add Bold Tags.vi"("Selection"=w460, "Value"=w461) -> ("Selection out"=w458:T12, "Value out"=w455:string)  [unwired: 8 in]
        n209 = property class="Str"(reference=w459, error in=w463, "Value"=w455, "Text.Selection"=w458) -> (error out=w453:errorcluster)  [unwired: 1 out]
        n210 = Bundle By Name(cluster=w457, "FP.VI Desc"=w455) -> (w456:T1)
      }
      frame "UI: Remove Bold Tags" {
        n211 = control-ref of="VI Description"() -> (w473:refnum<vi>)
        n212 = property class="Str"(reference=w473, error in=w465) -> (reference out=w470:refnum<vi>, error out=w474:errorcluster, "Value"=w472:string, "Text.Selection"=w471:T12)
        n213 = call "Remove Bold Tags.vi"("Selection"=w471, "Value"=w472) -> ("Selection out"=w469:T12, "Value out"=w466:string)  [unwired: 8 in]
        n214 = property class="Str"(reference=w470, error in=w474, "Value"=w466, "Text.Selection"=w469) -> (error out=w464:errorcluster)  [unwired: 1 out]
        n215 = Bundle By Name(cluster=w468, "FP.VI Desc"=w466) -> (w467:T1)
      }
      frame "UI: Focus Desc" {
        n216 = control-ref of="VI Description"() -> (w479:refnum<vi>)
        n217 = property class="Str"(reference=w479, error in=w480, "Key Focus"=TRUE, "Text.Selection Start"=u32 4294967295 ("Text.Selection:End")) -> (error out=w475:errorcluster)  [unwired: 1 out]
      }
      frame "UI: Format Desc" {
        n218 = control-ref of="VI Description"() -> (w486:refnum<vi>)
        n219 = Unbundle By Name(w483) -> ("Config.Format Bold Tags?"=w482:bool, "Desc Selection"=w481:T12)
        n220 = in-place {
          in-place-border: [w496] -> w488
          in-place-border: w487 -> [w495]
          in-place-border: w486 -> [w494]
          in-place-border: w485 -> [w493]
          in-place-border: w482 -> [w490]
          in-place-border: w481 -> [w489]
          n221 = in-place-cluster #10(w483) -> ("FP.VI Desc"=w492:string)
          n222 = case shown="\"Style\", Default" w493 {
            tunnel: [w497 w513] -> w496
            tunnel: w495 -> [w500 w512]
            tunnel: w494 -> [w499 w511]
            tunnel: w492 -> [_ w509]
            tunnel: [w506 w509] -> w491
            tunnel: w490 -> [w505 w510]
            tunnel: w489 -> [_ w508]
            frame "Tags" {
              n223 = call "Reset Plain Formatting.vi"("error in (no error)"=w500, "String Ref"=w499) -> ("error out"=w501:errorcluster, "String Ref out"=w498:refnum<vi>)  [unwired: 8 in]
              n224 = call "Find Bold Formatting.vi"("error in (no error)"=w501, "String Ref"=w498) -> ("error out"=w507:errorcluster, "Length"=w502:i32[], "Start"=w503:i32[], "String Ref out"=w504:refnum<vi>)  [unwired: 6 in]
              n225 = call "Replace Formatting with Tags.vi"("Set Value? (T)"=w505, "error in (no error)"=w507, "Length"=w502, "Start"=w503, "String Ref"=w504) -> ("error out"=w497:errorcluster, "New String"=w506:string)  [unwired: 4 in, 1 out]
            }
            frame "Style", Default {
              n226 = case shown="False" w510 {
                tunnel: [w514 w519] -> w513
                tunnel: w512 -> [w514 w518]
                tunnel: w511 -> [_ w517]
                tunnel: w509 -> [_ w516]
                tunnel: w508 -> [_ w515]
                frame False {
                }
                frame True {
                  n227 = call "Bold Description String.vi"("error in (no error)"=w518, "Selection"=w515, "String"=w516, "String Ref"=w517) -> ("error out"=w519:errorcluster)  [unwired: 7 in]
                }
              }
            }
          }
          n228 = in-place-cluster #10("FP.VI Desc"=w491) -> (w484:T1)
        }
      }
      frame "UI: Confirm" {
        n229 = case shown="\"Exit\"" w523 {
          tunnel: [w528 w547 w567 w586 w605 w627] -> w521
          tunnel: w526 -> [w537 w556 w575 w594 w613 w631]
          tunnel: w524 -> [w538 w557 w576 w595 w614 w630]
          tunnel: [w536 w555 w574 w593 w612 w631] -> w525
          tunnel: [w535 w554 w573 w592 w611 w630] -> w522
          tunnel: [w529 w548 w566 w585 w604 ""] -> w520
          frame "Save", Default {
            w531 = ""
            n230 = in-place {
              in-place-border: w537 -> [w545]
              in-place-border: [w543] -> w536
              in-place-border: [w541] -> w533
              in-place-border: [w540] -> w534
              n231 = in-place-cluster #11(w538) -> ("Config"=w546:T8)
              n232 = control-ref of="This VI"() -> (w539:refnum<vi>)
              n233 = call "Display Confirmation to User.vi"("Calling VI in"=w539, "Confirmation Type"=Confirmation_Type."Save", "error in (no error)"=w545, "Config"=w546) -> ("error out"=w543:errorcluster, "New Config?"=w541:bool, "OK?"=w540:bool, "Config out"=w544:T8)  [unwired: 4 in]
              n234 = in-place-cluster #11("Config"=w544) -> (w535:T1)
            }
            n235 = Select(t="Data: Write Config", s=w533, f=w531) -> (s? t:f=w529:string)
            n236 = Select(t="Macro: Save", s=w534, f=w531) -> (s? t:f=w528:string)
          }
          frame "Go Next" {
            w550 = ""
            n237 = in-place {
              in-place-border: w556 -> [w564]
              in-place-border: [w562] -> w555
              in-place-border: [w560] -> w552
              in-place-border: [w559] -> w553
              n238 = in-place-cluster #12(w557) -> ("Config"=w565:T8)
              n239 = control-ref of="This VI"() -> (w558:refnum<vi>)
              n240 = call "Display Confirmation to User.vi"("Calling VI in"=w558, "Confirmation Type"=Confirmation_Type."Save", "error in (no error)"=w564, "Config"=w565) -> ("error out"=w562:errorcluster, "New Config?"=w560:bool, "OK?"=w559:bool, "Config out"=w563:T8)  [unwired: 4 in]
              n241 = in-place-cluster #12("Config"=w563) -> (w554:T1)
            }
            n242 = Select(t="Data: Write Config", s=w552, f=w550) -> (s? t:f=w548:string)
            n243 = Select(t="Macro: Save >> Go Next", s=w553, f=w550) -> (s? t:f=w547:string)
          }
          frame "Revert" {
            w569 = ""
            n244 = in-place {
              in-place-border: w575 -> [w583]
              in-place-border: [w581] -> w574
              in-place-border: [w579] -> w571
              in-place-border: [w578] -> w572
              n245 = in-place-cluster #13(w576) -> ("Config"=w584:T8)
              n246 = control-ref of="This VI"() -> (w577:refnum<vi>)
              n247 = call "Display Confirmation to User.vi"("Calling VI in"=w577, "Confirmation Type"=Confirmation_Type."Revert", "error in (no error)"=w583, "Config"=w584) -> ("error out"=w581:errorcluster, "New Config?"=w579:bool, "OK?"=w578:bool, "Config out"=w582:T8)  [unwired: 4 in]
              n248 = in-place-cluster #13("Config"=w582) -> (w573:T1)
            }
            n249 = Select(t="Data: Write Config", s=w571, f=w569) -> (s? t:f=w566:string)
            n250 = Select(t="Macro: Revert", s=w572, f=w569) -> (s? t:f=w567:string)
          }
          frame "Save All" {
            w588 = ""
            n251 = in-place {
              in-place-border: w594 -> [w602]
              in-place-border: [w600] -> w593
              in-place-border: [w598] -> w590
              in-place-border: [w597] -> w591
              n252 = in-place-cluster #14(w595) -> ("Config"=w603:T8)
              n253 = control-ref of="This VI"() -> (w596:refnum<vi>)
              n254 = call "Display Confirmation to User.vi"("Calling VI in"=w596, "Confirmation Type"=Confirmation_Type."Save All", "error in (no error)"=w602, "Config"=w603) -> ("error out"=w600:errorcluster, "New Config?"=w598:bool, "OK?"=w597:bool, "Config out"=w601:T8)  [unwired: 4 in]
              n255 = in-place-cluster #14("Config"=w601) -> (w592:T1)
            }
            n256 = Select(t="Data: Write Config", s=w590, f=w588) -> (s? t:f=w585:string)
            n257 = Select(t="Macro: Save >> All", s=w591, f=w588) -> (s? t:f=w586:string)
          }
          frame "Revert All" {
            w607 = ""
            n258 = in-place {
              in-place-border: w613 -> [w621]
              in-place-border: [w619] -> w612
              in-place-border: [w617] -> w609
              in-place-border: [w616] -> w610
              n259 = in-place-cluster #15(w614) -> ("Config"=w622:T8)
              n260 = control-ref of="This VI"() -> (w615:refnum<vi>)
              n261 = call "Display Confirmation to User.vi"("Calling VI in"=w615, "Confirmation Type"=Confirmation_Type."Revert All", "error in (no error)"=w621, "Config"=w622) -> ("error out"=w619:errorcluster, "New Config?"=w617:bool, "OK?"=w616:bool, "Config out"=w620:T8)  [unwired: 4 in]
              n262 = in-place-cluster #15("Config"=w620) -> (w611:T1)
            }
            n263 = Select(t="Data: Write Config", s=w609, f=w607) -> (s? t:f=w604:string)
            n264 = Select(t="Macro: Revert >> All", s=w610, f=w607) -> (s? t:f=w605:string)
          }
          frame "Exit" {
            n265 = Unbundle By Name(w630) -> ("Config.Confirm Exit?"=w623:bool, "New VI Data"=w629:T3, "Saved VI Data"=w628:T3)
            n266 = Not Equal?(x=w629, y=w628) -> (x != y?=w624:bool)
            n267 = And(x=w623, y=w624) -> (x .and. y?=w625:bool)
            n268 = case "Unsaved changes AND need to confirm?" shown="False" w625 {
              tunnel: ["Macro: Exit" w633] -> w627
              frame False {
              }
              frame True {
                n269 = call <vilib>:"Three Button Dialog.vi"("Window Title (\"\")"="Confirm Exit" ("Window Title (\"\")"), "message"="You have unsaved changes. Save changes before closing?\n\n\nNote: This dialog can be deactivated in Options.") -> ("Which Button?"=w634:T22)  [unwired: 9 in]
                n270 = case shown="\"Left Button\"" w634 {
                  tunnel: ["Macro: Save >> Exit" "Macro: Exit" ""] -> w633
                  frame "Left Button" {
                  }
                  frame "Center Button" {
                  }
                  frame "Right Button", "Window Close" {
                  }
                }
              }
            }
          }
        }
        n271 = call "Enqueue Multiple States.vi"("State(s) at Front"=w521, "queue in"=w527, "State(s) at Back"=w520) -> ()  [unwired: 12 in, 1 out]
      }
      frame "UI: Edit Options" {
        n272 = in-place {
          in-place-border: w647 -> [w653]
          in-place-border: [w652] -> w646
          in-place-border: [w649] -> w643
          n273 = in-place-cluster #16(w645) -> ("Config"=w651:T8)
          n274 = call "Edit Options.vi"("error in (no error)"=w653, "Config"=w651) -> ("error out"=w652:errorcluster, "OK?"=w649:bool, "Config out"=w650:T8)  [unwired: 7 in]
          n275 = in-place-cluster #16("Config"=w650) -> (w644:T1)
        }
        n276 = Select(t="Data: Write Config\nUI: Initialize Menu\nUI: Format Item Names\nMacro: Load VI", s=w643, f="") -> (s? t:f=w640:string)
        n277 = call "Enqueue Multiple States.vi"("queue in"=w648, "State(s) at Back"=w640) -> ()  [unwired: 13 in, 1 out]
      }
      frame "UI: Add Custom Filter" {
        n278 = in-place {
          in-place-border: w661 -> [w667]
          in-place-border: [w666] -> w660
          in-place-border: [w663] -> w657
          n279 = in-place-cluster #17(w659) -> ("Filter"=w665:T9)
          n280 = call "Prompt for Custom Filter.vi"("error in (no error)"=w667, "Filter Info"=w665) -> ("error out"=w666:errorcluster, "OK?"=w663:bool, "Filter Info out"=w664:T9)  [unwired: 7 in]
          n281 = in-place-cluster #17("Filter"=w664) -> (w658:T1)
        }
        n282 = Select(t="UI: Menu Selection >> FILTER_Custom_Do", s=w657, f="") -> (s? t:f=w654:string)
        n283 = call "Enqueue Multiple States.vi"("queue in"=w662, "State(s) at Back"=w654) -> ()  [unwired: 13 in, 1 out]
      }
      frame "---------- Macro ----------" {
        # "Do not put any code in this frame.\n(It is a separator no-op. You can make a copy of this frame to create a new Macro frame)"
      }
      frame "Macro: Initialize" {
        w670 = "Data: Initialize\nInitialize Core Data\nData: Bundle Refs\nData: Read Config\nUI: Initialize\nUI: Interlocks\nUI: Front Panel State >> Open\nUI: Initialize Menu"  # Data: Initialize Initialize Core Data Data: Bundle Refs Data: Read Config UI: Initialize UI: Interlocks UI: Front Panel State >> Open UI: Initialize Menu
        # "Initialization Macro\n(This is called once, when the VI starts)"
        n284 = call "Enqueue Multiple States.vi"("State(s) at Front"=w670, "queue in"=w671) -> ()  [unwired: 13 in, 1 out]
      }
      frame "Macro: Load VI" {
        n285 = call "Enqueue Multiple States.vi"("State(s) at Front"="UI: Panel Updates >> Defer\nData: Update >> All Ctls\nUI: Display Data\nUI: Format Desc\nUI: Panel Updates >> Undefer\nUI: Interlocks", "queue in"=w675) -> ()  [unwired: 13 in, 1 out]
      }
      frame "Macro: Load Recent Source" {
        n286 = Search/Split String(string=w679, search string/char (-)="_") -> (substring before match=w681:string)  [unwired: 1 in, 2 out]
        n287 = Format Into String(format string="UI: Cursor Set >> Busy\nData: Update >> Reset Listbox\nData: Update >> %s\nData: Update >> %s Config\nData: Load VIs\nData: Write Config\nUI: Initialize Menu\nData: Filter/Sort VIs\nMacro: Load VI\nUI: Format Item Names\nUI: Cursor Set >> Idle", w679, w681) -> (resulting string=w678:string)  [unwired: 2 in, 1 out]
        n288 = call "Enqueue Multiple States.vi"("State(s) at Front"=w678, "queue in"=w683) -> ()  [unwired: 13 in, 1 out]
      }
      frame "Macro: Revert" {
        n289 = case shown="\"\", Default" w688 {
          tunnel: ["Data: Revert Current\nUI: Format Item Names\nMacro: Load VI" "Data: Revert All\nUI: Format Item Names\nMacro: Load VI"] -> w689
          frame "", Default {
          }
          frame "All" {
          }
        }
        n290 = call "Enqueue Multiple States.vi"("State(s) at Front"=w689, "queue in"=w690) -> ()  [unwired: 13 in, 1 out]
      }
      frame "Macro: Save" {
        n291 = case shown="\"All\"" w695 {
          tunnel: ["UI: Cursor Set >> Busy\nData: Save Current\nUI: Format Item Names\nUI: Interlocks\nUI: Cursor Set >> Idle" "UI: Cursor Set >> Busy\nData: Save Current\nUI: Format Item Names\nUI: Interlocks\nData: Update >> Inc Index\nMacro: Load VI\nUI: Cursor Set >> Idle\nUI: Focus Desc" "UI: Cursor Set >> Busy\nData: Save All\nUI: Format Item Names\nUI: Interlocks\nUI: Cursor Set >> Idle" "UI: Cursor Set >> Busy\nData: Save All\nUI: Format Item Names\nUI: Interlocks\nUI: Cursor Set >> Idle\nMacro: Exit"] -> w696
          frame "", Default {
          }
          frame "Go Next" {
          }
          frame "All" {
          }
          frame "Exit" {
          }
        }
        n292 = call "Enqueue Multiple States.vi"("State(s) at Front"=w696, "queue in"=w697) -> ()  [unwired: 13 in, 1 out]
      }
      frame "Macro: Exit" {
        # "#Todo:"
        # "Exit Macro\n(This is called once, when the VI exits)"
        n293 = Unbundle By Name(w715) -> ("Core.Close Panel on Exit?"=w714:bool, "FP Refs.VI Tree"=w703:refnum<vi>)
        n294 = Generate User Event(user event=w706, event data cluster=FALSE ("event data"), error in=w716) -> (error out=w707:errorcluster)  [unwired: 1 in, 1 out]
        n295 = invoke class="VI" method="Default Vals.Reinit All"() -> ()  [unwired: 3 in, 3 out]
        n296 = property class="Tree (strict)"(reference=w703, "ColHdrString"=string[] [] ("Column Header Strings[]")) -> ()  [unwired: 1 in, 2 out]
        n297 = invoke class="Tree (strict)" method="Edit Tree Items.Delete"(reference=w703) -> ()  [unwired: 4 in, 5 out]
        n298 = property on="VI Tree" class="Tree (strict)"("TopLeft"=T19 {"Node"="", "Column"=0} ("Top Left Visible Cell")) -> ()  [unwired: 2 in, 2 out]
        n299 = Select(t="UI: Front Panel State >> Close\n", s=w714, f="") -> (s? t:f=w710:string)
        n300 = Concatenate Strings(w710, "Data: Cleanup\nExit") -> (w708:string)
        n301 = call "Enqueue Multiple States.vi"("State(s) at Front"=w708, "queue in"=w711) -> ()  [unwired: 13 in, 1 out]
      }
    }
  }
  n302 = while "Producer Loop" {
    shift-right: [w720] -> w9
    shift-left: w15 -> [w724]
    tunnel: w3 -> [w717]
    tunnel: w11 -> [w723]
    tunnel: [w718] -> w7
    stop <- w722 stop-if-true
    # "executes when the state queue is empty"
    n303 = event shown="[6] <Enqueue Macro?>: User Event" {
      selector: w717 -> [_ _ _ _ _ _ _]
      dyn-events: _ -> [_ _ _ _ _ _ _]
      timeout: _ -> [_ _ _ _ _ _ _]
      tunnel: [w726 w738 w750 w754 w760 w767 w775] -> w721
      tunnel: w724 -> [w726 w739 w750 w754 w760 w767 w775]
      tunnel: w723 -> [w727 w737 w751 w755 w759 w764 w774]
      tunnel: [w728 w740 w752 w756 w758 w763 w773] -> w719
      tunnel: [_ _ _ _ _ _ TRUE] -> w722
      event "Add Copyright": Value Change {
        n304 = event-data() -> ()  [unwired: 1 in, 6 out]
        n305 = call "Enqueue Multiple States.vi"("queue in"=w727, "State(s) at Back"="Data: Add Copyright\nUI: Format Item Names\nUI: Display Data") -> ("queue out"=w728:refnum<queue>)  [unwired: 13 in]
      }
      event "VI Tree", "Help Path", "Help Tag", "VI Description", "Controls", "Window Title", "Same Title as VI?": Value Change {
        n306 = event-data() -> ("CtlRef"=w735:refnum<vi>, "NewVal"=w729:variant)  [unwired: 1 in]
        n307 = property class="Ctl"(reference=w735) -> ("Label.Text"=w731:string)  [unwired: 1 in, 2 out]
        n308 = case shown="\"VI Tree\"" w731 {
          tunnel: ["" "Macro: Load VI" "Data: Value Changed\nUI: Format Item Names\nUI: Interlocks" "Data: Value Changed\nUI: Format Item Names\nUI: Interlocks" "Data: Update >> Selection\nData: Value Changed\nUI: Format Item Names\nUI: Format Desc\nUI: Interlocks" "Data: Change Controls\nUI: Format Item Names\nUI: Interlocks" "Data: Value Changed\nUI: Format Item Names\nUI: Interlocks" "Data: Value Changed\nUI: Format Item Names\nUI: Interlocks"] -> w730
          frame Default {
          }
          frame "VI Tree" {
          }
          frame "Help Path" {
          }
          frame "Help Tag" {
          }
          frame "VI Description" {
          }
          frame "Controls" {
          }
          frame "Window Title" {
          }
          frame "Same Title as VI?" {
          }
        }
        n309 = Format Into String(format string="Data: Update >> %s", w731) -> (resulting string=w733:string)  [unwired: 2 in, 1 out]
        n310 = Bundle(w733, "NewVal"=w729) -> (w732:cluster{string, "NewVal":variant})  [unwired: 1 in]
        n311 = Enqueue Element(queue=w737, element=w732, error in (no error)=w739) -> (queue out=w736:refnum<queue>, error out=w738:errorcluster)  [unwired: 1 in, 1 out]
        n312 = call "Enqueue Multiple States.vi"("queue in"=w736, "State(s) at Back"=w730) -> ("queue out"=w740:refnum<queue>)  [unwired: 13 in]
      }
      event "Set all VIs": Value Change {
        n313 = event-data() -> ()  [unwired: 1 in, 6 out]
        n314 = call "Enqueue Multiple States.vi"("queue in"=w751, "State(s) at Back"="Data: Set All VIs\nUI: Format Item Names") -> ("queue out"=w752:refnum<queue>)  [unwired: 13 in]
      }
      event "VI Tree": Double Click {
        n315 = event-data() -> ()  [unwired: 1 in, 10 out]
        n316 = call "Enqueue Multiple States.vi"("queue in"=w755, "State(s) at Back"="UI: Open VI") -> ("queue out"=w756:refnum<queue>)  [unwired: 13 in]
      }
      event Menu Selection (User) {
        n317 = event-data() -> ("ItemTag"=w761:string)  [unwired: 1 in]
        n318 = Format Into String(format string="UI: Menu Selection >> %s", w761) -> (resulting string=w757:string)  [unwired: 2 in, 1 out]
        n319 = call "Enqueue Multiple States.vi"("queue in"=w759, "State(s) at Back"=w757) -> ("queue out"=w758:refnum<queue>)  [unwired: 13 in]
      }
      event Panel Close? {
        # "Discard the event because we'll close the front panel ourselves in Macro: Exit"
        # "Close Panel button (pressed) Event\n(this executes Macro: Exit to terminate the VI)"
        n320 = event-data() -> ()  [unwired: 1 in, 1 out]
        n321 = event-data("Discard?"=TRUE) -> ()  [unwired: 1 in, 1 out]
        n322 = call "Enqueue Multiple States.vi"("State(s) at Front"="UI: Confirm >> Exit", "queue in"=w764) -> ("queue out"=w763:refnum<queue>)  [unwired: 13 in]
      }
      event User Event {
        # "\"Exit\" Dynamic Event registered\n(this executes Macro: Exit to terminate the VI)"
        n323 = event-data() -> ("Enqueue Macro?"=w771:bool)  [unwired: 1 in]
        n324 = Select(t="Macro: Exit", s=w771, f="") -> (s? t:f=w768:string)
        n325 = call "Enqueue Multiple States.vi"("State(s) at Front"=w768, "queue in"=w774) -> ("queue out"=w773:refnum<queue>)  [unwired: 13 in]
      }
    }
    n326 = call "Producer Loop Guard Clause.vi"("error in (no error)"=w721, "queue in"=w719) -> ("error out"=w720:errorcluster, "queue out"=w718:refnum<queue>)  [unwired: 8 in]
  }
  n327 = Merge Errors(w9, w10) -> (w8:errorcluster)
  n328 = Release Queue(queue=w7, error in (no error)=w8) -> ()  [unwired: 1 in, 3 out]
